vi "单数据解析_new.vi"(0 "Data1":u8, 1 "Data2":u8, 2 "Data3":u8, 3 "Data4":u8, 4 "Data5":u8, 5 "Data6":u8, 6 "Data7":u8, 7 "Data8":u8, 8 "ID":i32 format="%x", 9 "选项卡数值":enum32{"单体电压", "单体温度", "单体内阻", "单体SOC"}(ring)) -> (20 "位置":i32[](array[numeric]), 22 "数据":dbl[](array[numeric]), 24 "放电均衡":i32[](array[numeric]), 25 "充电均衡":i32[](array[numeric]), 26 "PF":i32, 27 "均衡故障":dbl[](array[numeric]))   [LabVIEW 2013]
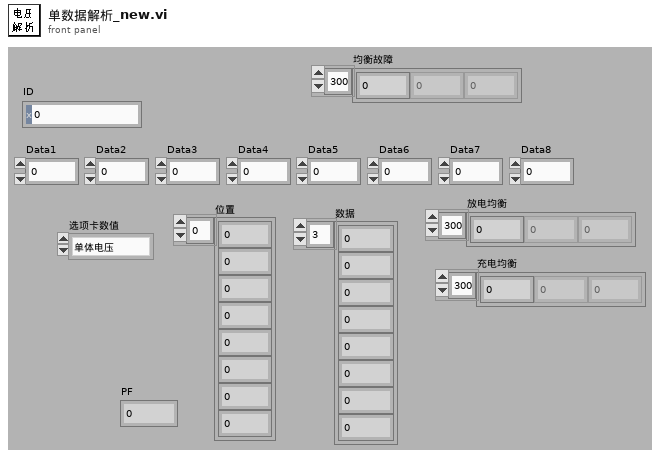
[diagram p1: front panel]
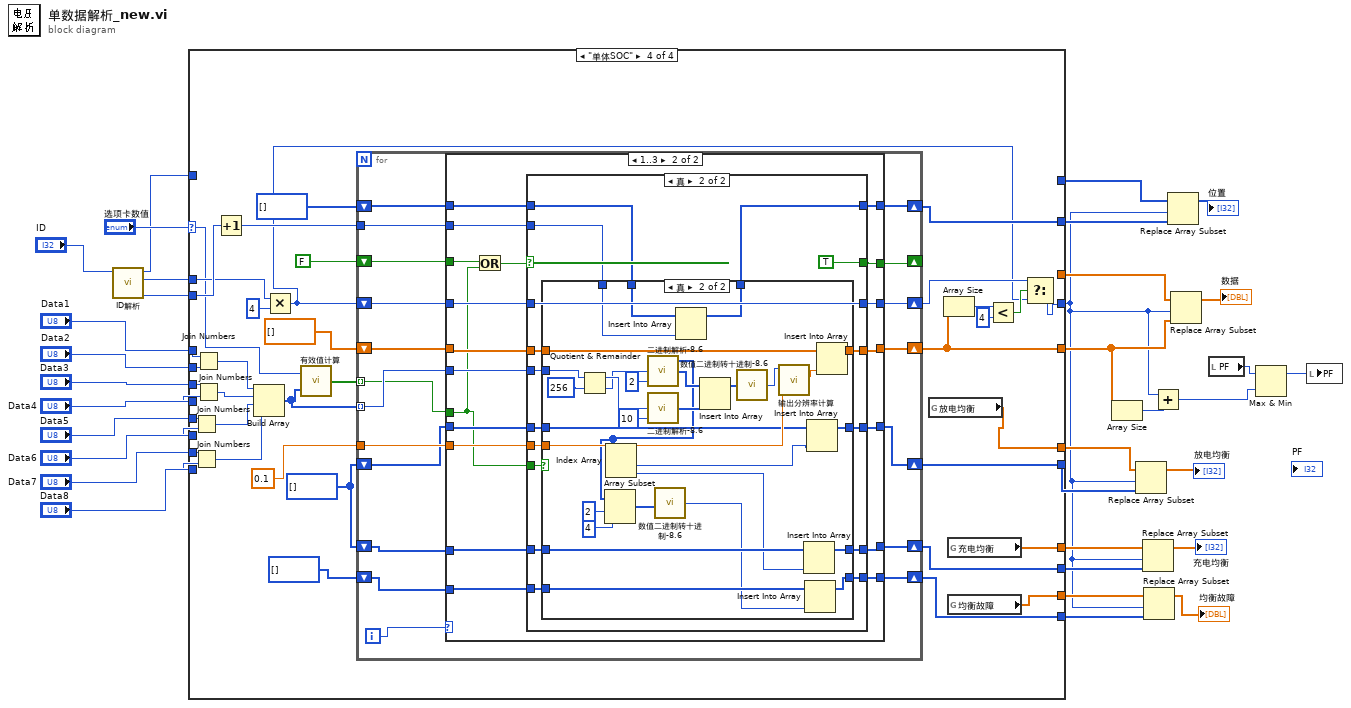
[diagram p0: block diagram]
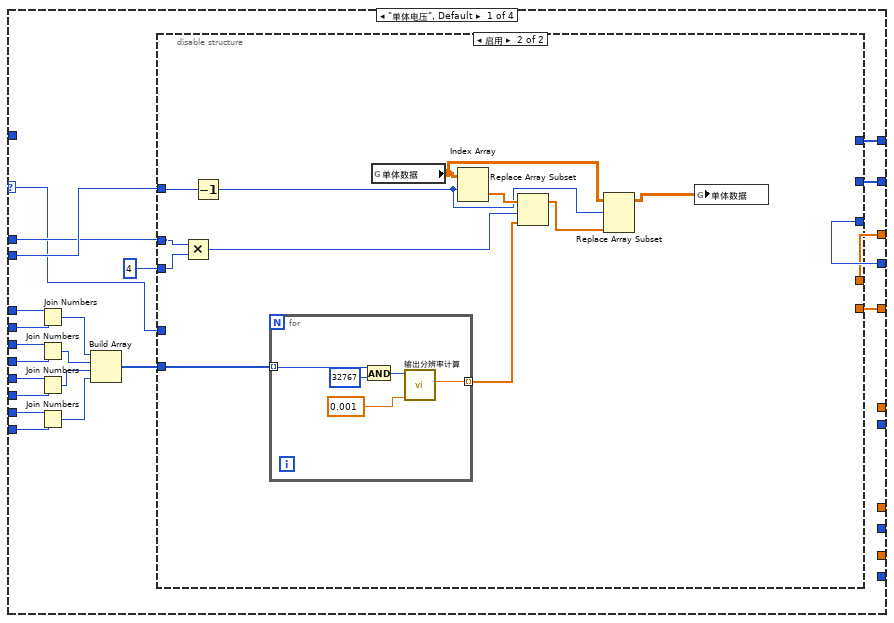
[diagram p2: hidden frame]
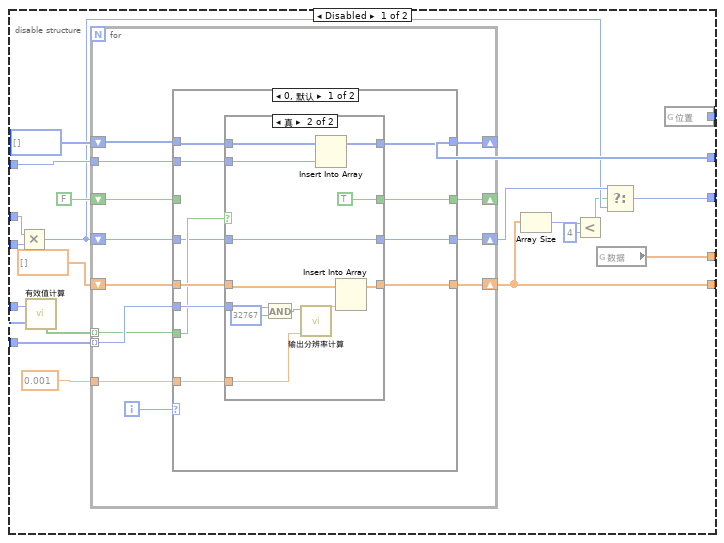
[diagram p3: hidden frame]
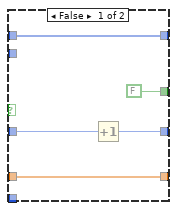
[diagram p4: hidden frame]
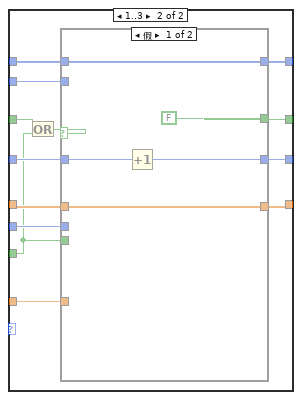
[diagram p5: hidden frame]
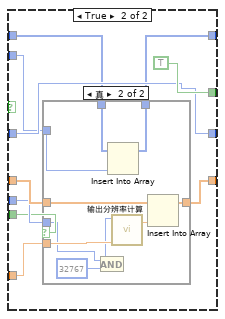
[diagram p6: hidden frame]
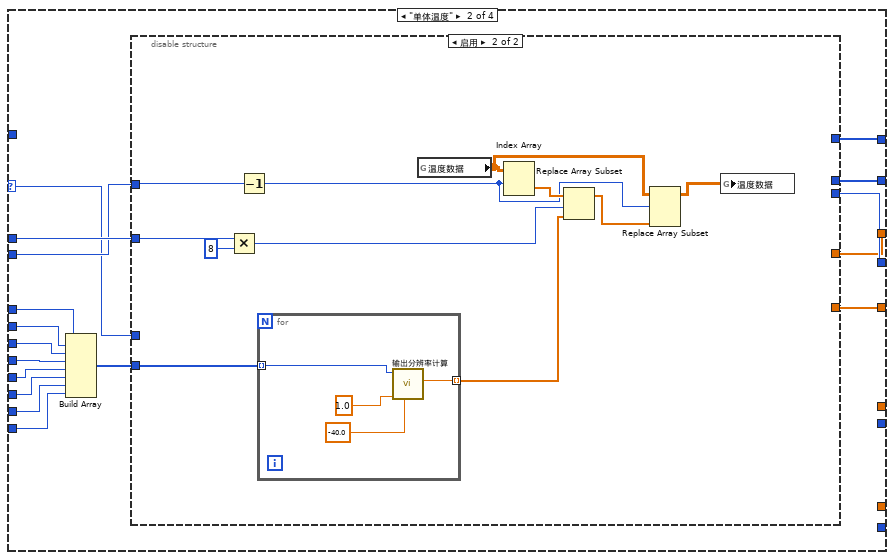
[diagram p8: hidden frame]
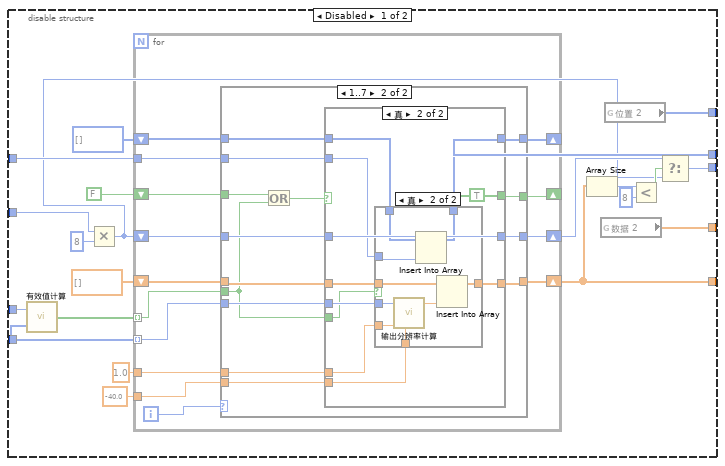
[diagram p9: hidden frame]
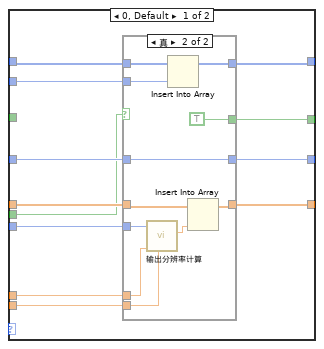
[diagram p10: hidden frame]
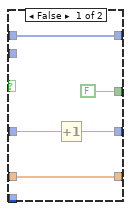
[diagram p11: hidden frame]
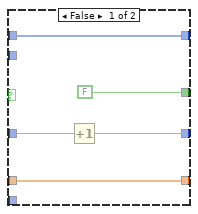
[diagram p12: hidden frame]
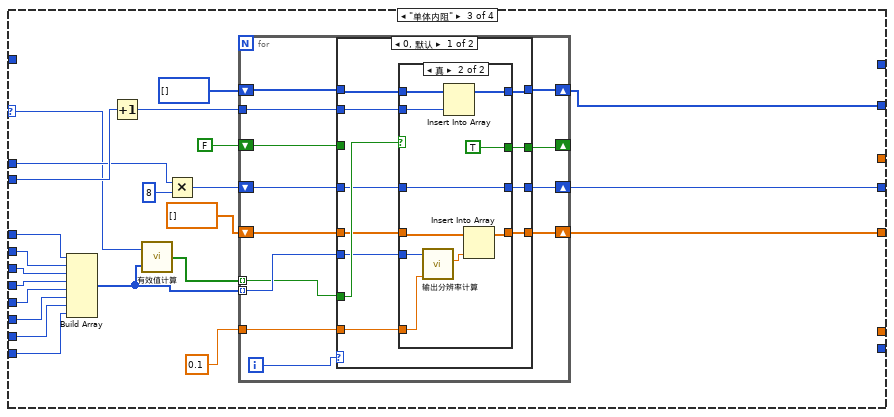
[diagram p14: hidden frame]
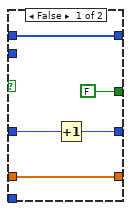
[diagram p15: hidden frame]
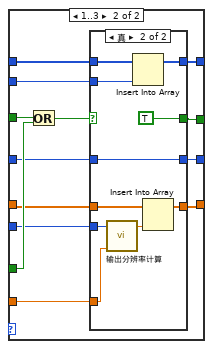
[diagram p16: hidden frame]
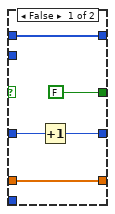
[diagram p17: hidden frame]
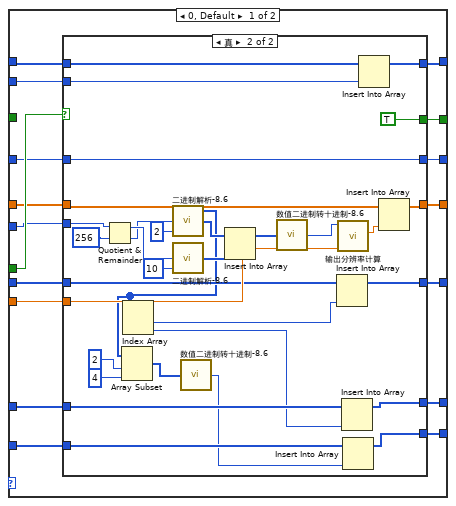
[diagram p18: hidden frame]
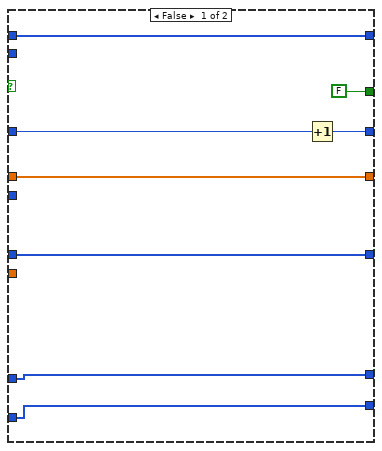
[diagram p19: hidden frame]
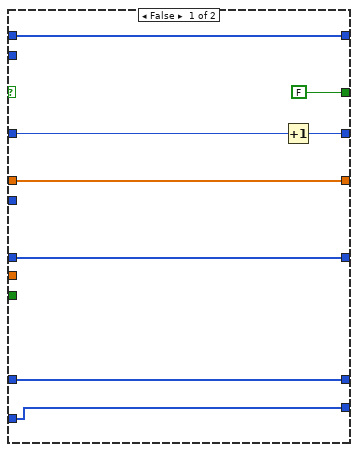
[diagram p20: hidden frame]
diagram:
  n1 = call "ID解析.vi"("ID"="ID") -> ("SA(4)"=w18:i32, "PF(2)"=w17:i32, "PDU(1)"=w29:i32)  [unwired: 8 out]
  n2 = case shown="\"单体SOC\"" "选项卡数值" {
    selector: "选项卡数值" -> [w34 w173 w310 w400]
    tunnel: "Data2" -> [w55 w187 w318 w429]
    tunnel: "Data1" -> [w54 w188 w319 w428]
    tunnel: "Data3" -> [w53 w186 w317 w427]
    tunnel: "Data4" -> [w52 w185 w316 w426]
    tunnel: "Data5" -> [w51 w184 w315 w425]
    tunnel: "Data7" -> [w50 w182 w313 w423]
    tunnel: "Data8" -> [w49 w181 w312 w422]
    tunnel: "Data6" -> [w48 w183 w314 w424]
    tunnel: [w46 w178 w328 w406] -> w3
    tunnel: [w47 w189 w323 w431] -> w33
    tunnel: [w45 w180 w322 w410] -> w5
    tunnel: w18 -> [w44 w177 w321 w430]
    tunnel: w17 -> [w43 w179 w320 w408]
    tunnel: [_ _ _ w417] -> w14
    tunnel: w29 -> [_ _ _ _]
    tunnel: [w37 w176 _ _] -> w16
    tunnel: [w36 w175 _ _] -> w15
    tunnel: [_ _ _ w416] -> w13
    tunnel: [_ _ _ w415] -> w12
    tunnel: [_ _ _ w405] -> w9
    tunnel: [_ _ _ w403] -> w8
    tunnel: [_ _ _ w402] -> w7
    frame "单体电压", Default {
      n3 = Join Numbers(hi=w54, lo=w55) -> ((hi.lo)=w41:u16)
      n4 = Join Numbers(hi=w53, lo=w52) -> ((hi.lo)=w40:u16)
      n5 = Join Numbers(hi=w51, lo=w48) -> ((hi.lo)=w39:u16)
      n6 = Join Numbers(hi=w50, lo=w49) -> ((hi.lo)=w38:u16)
      n7 = Build Array(w41, w40, w39, w38) -> (w35:u16[])
      n8 = disable-structure shown="启用" {
        disable-tunnel: [w75 _] -> w47
        disable-tunnel: [w74 _] -> w46
        disable-tunnel: [w73 _] -> w45
        disable-tunnel: w44 -> [w72 w166]
        disable-tunnel: w43 -> [w71 w164]
        disable-tunnel: 4 ("y") -> [w70 w163]
        disable-tunnel: [w60 _] -> w37
        disable-tunnel: [w59 _] -> w36
        disable-tunnel: w35 -> [w58 w167]
        disable-tunnel: w34 -> [w56 _]
        frame Disabled {
          n9 = Multiply(x=w71, y=w70) -> (x*y=w64:i32)
          n10 = call "有效值计算.vi"("数组"=w58, "选项卡数值"=w56) -> ("有效位"=w57:bool[])
          n11 = for {
            tunnel: w58 -> [w85] mode=indexing
            shift-right: [w86] -> w73
            shift-left: dbl[] [] -> [w87]
            tunnel: 0.001 ("分辨率") -> [w84]
            shift-right: [w82] -> w75
            shift-left: i32[] [] -> [w83]
            tunnel: w72 -> [w81]
            shift-right: [w80] -> _
            shift-left: FALSE -> [w79]
            shift-right: [w77] -> w65
            shift-left: w64 -> [w78]
            tunnel: w57 -> [w76] mode=indexing
            i -> [w88]
            n12 = case shown="0, 默认" w88 {
              tunnel: w76 -> [w91 w117]
              tunnel: [w99 w129] -> w80
              tunnel: w87 -> [w98 w128]
              tunnel: [w97 w127] -> w86
              tunnel: w85 -> [w96 w126]
              tunnel: w84 -> [w95 w125]
              tunnel: w83 -> [w94 w124]
              tunnel: [w93 w123] -> w82
              tunnel: w81 -> [w92 w122]
              tunnel: w79 -> [_ w118]
              tunnel: w78 -> [w90 w121]
              tunnel: [w89 w120] -> w77
              frame 0, Default {
                n13 = case shown="真" w91 {
                  tunnel: [FALSE TRUE] -> w99
                  tunnel: w98 -> [w103 w115]
                  tunnel: [w103 w114] -> w97
                  tunnel: w96 -> [_ w107]
                  tunnel: w95 -> [_ w112]
                  tunnel: w94 -> [w102 w111]
                  tunnel: [w102 w110] -> w93
                  tunnel: w92 -> [_ w109]
                  tunnel: w90 -> [w101 w108]
                  tunnel: [w100 w108] -> w89
                  frame False {
                    n14 = Increment(x=w101) -> (x+1=w100:i32)
                  }
                  frame True {
                    n15 = And(x=w107, y=u16 32767) -> (x .and. y?=w105:u16)
                    n16 = call "输出分辨率计算.vi"("分辨率"=w112, "数值 2"=w105) -> ("输出2"=w113:dbl)  [unwired: 4 in, 5 out]
                    n17 = Insert Into Array(array=w111, new element=w109) -> (w110:i32[])  [unwired: 1 in]
                    n18 = Insert Into Array(array=w115, new element=w113) -> (w114:dbl[])  [unwired: 1 in]
                  }
                }
              }
              frame 1..3 {
                n19 = Or(x=w118, y=w117) -> (x .or. y?=w119:bool)
                n20 = case shown="假" w119 {
                  tunnel: [FALSE TRUE] -> w129
                  tunnel: w128 -> [w134 w143]
                  tunnel: [w134 w142] -> w127
                  tunnel: w126 -> [_ w141]
                  tunnel: w125 -> [_ w140]
                  tunnel: w124 -> [w133 w136]
                  tunnel: [w133 w135] -> w123
                  tunnel: w122 -> [_ w137]
                  tunnel: w121 -> [w131 w139]
                  tunnel: [w130 w139] -> w120
                  tunnel: w117 -> [_ w138]
                  frame False {
                    n21 = Increment(x=w131) -> (x+1=w130:i32)
                  }
                  frame True {
                    n22 = case shown="真" w138 {
                      tunnel: w143 -> [w146 w156]
                      tunnel: [w146 w155] -> w142
                      tunnel: w141 -> [_ w148]
                      tunnel: w140 -> [_ w154]
                      tunnel: w137 -> [_ w152]
                      tunnel: w136 -> [w145 w151]
                      tunnel: [w145 w150] -> w135
                      frame False {
                      }
                      frame True {
                        n23 = And(x=w148, y=u16 32767) -> (x .and. y?=w147:u16)
                        n24 = Insert Into Array(array=w151, new element=w152) -> (w150:i32[])  [unwired: 1 in]
                        n25 = call "输出分辨率计算.vi"("分辨率"=w154, "数值 2"=w147) -> ("输出2"=w153:dbl)  [unwired: 4 in, 5 out]
                        n26 = Insert Into Array(array=w156, new element=w153) -> (w155:dbl[])  [unwired: 1 in]
                      }
                    }
                  }
                }
              }
            }
          }
          n27 = Array Size(array=w73) -> (size(s)=w63:i32)
          n28 = Less?(x=w63, y=4) -> (x < y?=w61:bool)
          n29 = global read "单体信息全局.vi" "数据"() -> (w59:dbl[])
          n30 = Select(t=w65, s=w61, f=w64) -> (s? t:f=w74:i32)
          n31 = global read "单体信息全局.vi" "位置"() -> (w60:i32[])
        }
        frame Enabled {
          n32 = Multiply(x=w164, y=w163) -> (x*y=w162:i32)
          n33 = Decrement(x=w166) -> (x-1=w159:i32)
          n34 = for {
            tunnel: w167 -> [w172] mode=indexing
            tunnel: [w168] -> w161 mode=indexing
            n35 = And(x=w172, y=u16 32767) -> (x .and. y?=w170:u16)
            n36 = call "输出分辨率计算.vi"("分辨率"=0.001, "数值 2"=w170) -> ("输出2"=w168:dbl)  [unwired: 4 in, 5 out]
          }
          n37 = global read "单体信息全局.vi" "单体数据"() -> (w160:dbl[][])
          n38 = Index Array(array=w160, index (row)=w159) -> (element=w165:dbl[])  [unwired: 1 in]
          n39 = Replace Array Subset(array=w165, new element=w161, index=w162) -> (w158:dbl[])
          n40 = Replace Array Subset(array=w160, new element=w158, index (row)=w159) -> (w157:dbl[][])  [unwired: 1 in]
          n41 = global write "单体信息全局.vi" "单体数据"(w157) -> ()
        }
      }
    }
    frame "单体温度" {
      n42 = Build Array(w188, w187, w186, w185, w184, w183, w182, w181) -> (w174:u8[])
      n43 = disable-structure shown="启用" {
        disable-tunnel: [w210 _] -> w189
        disable-tunnel: [w209 _] -> w180
        disable-tunnel: w179 -> [w208 w296]
        disable-tunnel: [w207 _] -> w178
        disable-tunnel: w177 -> [w206 w294]
        disable-tunnel: [w194 _] -> w176
        disable-tunnel: [w193 _] -> w175
        disable-tunnel: w174 -> [w192 w298]
        disable-tunnel: w173 -> [w190 _]
        frame Disabled {
          n44 = call "有效值计算.vi"("数组"=w192, "选项卡数值"=w190) -> ("有效位"=w191:bool[])
          n45 = Multiply(x=w208, y=8) -> (x*y=w195:i32)
          n46 = for {
            tunnel: w192 -> [w217] mode=indexing
            shift-right: [w222] -> w196
            shift-left: w195 -> [w223]
            shift-right: [w221] -> _
            shift-left: FALSE -> [w220]
            shift-right: [w218] -> w209
            shift-left: dbl[] [] -> [w219]
            tunnel: 1.0 ("分辨率") -> [w216]
            shift-right: [w214] -> w210
            shift-left: i32[] [] -> [w215]
            tunnel: w206 -> [w213]
            tunnel: -40.0 ("分辨率") -> [w212]
            tunnel: w191 -> [w211] mode=indexing
            i -> [w224]
            n47 = case shown="1..7" w224 {
              tunnel: w223 -> [w236 w264]
              tunnel: [w235 w263] -> w222
              tunnel: [w234 w262] -> w221
              tunnel: w220 -> [_ w265]
              tunnel: w219 -> [w233 w261]
              tunnel: [w232 w260] -> w218
              tunnel: w217 -> [w231 w259]
              tunnel: w216 -> [w230 w258]
              tunnel: w215 -> [w229 w257]
              tunnel: [w228 w256] -> w214
              tunnel: w213 -> [w227 w255]
              tunnel: w212 -> [w226 w254]
              tunnel: w211 -> [w225 w253]
              frame 0, Default {
                n48 = case shown="真" w225 {
                  tunnel: w236 -> [w240 w252]
                  tunnel: [w239 w252] -> w235
                  tunnel: [FALSE TRUE] -> w234
                  tunnel: w233 -> [w238 w250]
                  tunnel: [w238 w249] -> w232
                  tunnel: w231 -> [_ w248]
                  tunnel: w230 -> [_ w246]
                  tunnel: w229 -> [w237 w245]
                  tunnel: [w237 w244] -> w228
                  tunnel: w227 -> [_ w243]
                  tunnel: w226 -> [_ w242]
                  frame False {
                    n49 = Increment(x=w240) -> (x+1=w239:i32)
                  }
                  frame True {
                    n50 = call "输出分辨率计算.vi"("偏移量"=w242, "分辨率"=w246, "数值 2"=w248) -> ("输出2"=w247:dbl)  [unwired: 3 in, 5 out]
                    n51 = Insert Into Array(array=w245, new element=w243) -> (w244:i32[])  [unwired: 1 in]
                    n52 = Insert Into Array(array=w250, new element=w247) -> (w249:dbl[])  [unwired: 1 in]
                  }
                }
              }
              frame 1..7 {
                n53 = Or(x=w265, y=w253) -> (x .or. y?=w266:bool)
                n54 = case shown="真" w266 {
                  tunnel: w264 -> [w271 w282]
                  tunnel: [w270 w282] -> w263
                  tunnel: [FALSE TRUE] -> w262
                  tunnel: w261 -> [w268 w280]
                  tunnel: [w268 w279] -> w260
                  tunnel: w259 -> [_ w278]
                  tunnel: w258 -> [_ w277]
                  tunnel: w257 -> [w267 w274]
                  tunnel: [w267 w273] -> w256
                  tunnel: w255 -> [_ w275]
                  tunnel: w254 -> [_ w276]
                  tunnel: w253 -> [_ w272]
                  frame False {
                    n55 = Increment(x=w271) -> (x+1=w270:i32)
                  }
                  frame True {
                    n56 = case shown="真" w272 {
                      tunnel: w280 -> [w284 w293]
                      tunnel: [w284 w292] -> w279
                      tunnel: w278 -> [_ w291]
                      tunnel: w277 -> [_ w290]
                      tunnel: w276 -> [_ w289]
                      tunnel: w275 -> [_ w287]
                      tunnel: w274 -> [w283 w286]
                      tunnel: [w283 w285] -> w273
                      frame False {
                      }
                      frame True {
                        n57 = call "输出分辨率计算.vi"("偏移量"=w289, "分辨率"=w290, "数值 2"=w291) -> ("输出2"=w288:dbl)  [unwired: 3 in, 5 out]
                        n58 = Insert Into Array(array=w286, new element=w287) -> (w285:i32[])  [unwired: 1 in]
                        n59 = Insert Into Array(array=w293, new element=w288) -> (w292:dbl[])  [unwired: 1 in]
                      }
                    }
                  }
                }
              }
            }
          }
          n60 = Array Size(array=w209) -> (size(s)=w199:i32)
          n61 = global read "单体信息全局.vi" "数据 2"() -> (w193:dbl[])
          n62 = global read "单体信息全局.vi" "位置 2"() -> (w194:i32[])
          n63 = Less?(x=w199, y=8) -> (x < y?=w197:bool)
          n64 = Select(t=w196, s=w197, f=w195) -> (s? t:f=w207:i32)
        }
        frame Enabled {
          n65 = Multiply(x=w296, y=8) -> (x*y=w303:i32)
          n66 = Decrement(x=w294) -> (x-1=w300:i32)
          n67 = for {
            tunnel: w298 -> [w305] mode=indexing
            tunnel: [w307] -> w302 mode=indexing
            n68 = call "输出分辨率计算.vi"("偏移量"=sgl -40.0, "分辨率"=1.0, "数值 2"=w305) -> ("输出2"=w307:dbl)  [unwired: 3 in, 5 out]
          }
          n69 = global read "单体信息全局.vi" "温度数据"() -> (w301:sgl[][])
          n70 = Index Array(array=w301, index (row)=w300) -> (element=w304:sgl[])  [unwired: 1 in]
          n71 = Replace Array Subset(array=w304, new element=w302, index=w303) -> (w299:sgl[])
          n72 = Replace Array Subset(array=w301, new element=w299, index (row)=w300) -> (w297:sgl[][])  [unwired: 1 in]
          n73 = global write "单体信息全局.vi" "温度数据"(w297) -> ()
        }
      }
    }
    frame "单体内阻" {
      n74 = Build Array(w319, w318, w317, w316, w315, w314, w313, w312) -> (w311:u8[])
      n75 = Increment(x=w321) -> (x+1=w325:i32)
      n76 = call "有效值计算.vi"("数组"=w311, "选项卡数值"=w310) -> ("有效位"=w309:bool[])
      n77 = Multiply(x=w320, y=8) -> (x*y=w330:i32)
      n78 = for {
        tunnel: w311 -> [w337] mode=indexing
        shift-right: [w342] -> w328
        shift-left: w330 -> [w343]
        shift-right: [w341] -> _
        shift-left: FALSE -> [w340]
        shift-right: [w338] -> w322
        shift-left: dbl[] [] -> [w339]
        tunnel: 0.1 ("分辨率") -> [w336]
        shift-right: [w334] -> w323
        shift-left: i32[] [] -> [w335]
        tunnel: w325 -> [w333]
        tunnel: w309 -> [w332] mode=indexing
        i -> [w344]
        n79 = case shown="0, 默认" w344 {
          tunnel: w332 -> [w355 w381]
          tunnel: w343 -> [w354 w380]
          tunnel: [w353 w379] -> w342
          tunnel: [w352 w378] -> w341
          tunnel: w340 -> [_ w382]
          tunnel: w339 -> [w351 w377]
          tunnel: [w350 w376] -> w338
          tunnel: w337 -> [w349 w375]
          tunnel: w336 -> [w348 w374]
          tunnel: w335 -> [w347 w373]
          tunnel: [w346 w372] -> w334
          tunnel: w333 -> [w345 w371]
          frame 0, Default {
            n80 = case shown="真" w355 {
              tunnel: w354 -> [w359 w370]
              tunnel: [w358 w370] -> w353
              tunnel: [FALSE TRUE] -> w352
              tunnel: w351 -> [w357 w368]
              tunnel: [w357 w367] -> w350
              tunnel: w349 -> [_ w366]
              tunnel: w348 -> [_ w364]
              tunnel: w347 -> [w356 w363]
              tunnel: [w356 w362] -> w346
              tunnel: w345 -> [_ w361]
              frame False {
                n81 = Increment(x=w359) -> (x+1=w358:i32)
              }
              frame True {
                n82 = call "输出分辨率计算.vi"("分辨率"=w364, "数值 2"=w366) -> ("输出2"=w365:dbl)  [unwired: 4 in, 5 out]
                n83 = Insert Into Array(array=w363, new element=w361) -> (w362:i32[])  [unwired: 1 in]
                n84 = Insert Into Array(array=w368, new element=w365) -> (w367:dbl[])  [unwired: 1 in]
              }
            }
          }
          frame 1..3 {
            n85 = Or(x=w382, y=w381) -> (x .or. y?=w383:bool)
            n86 = case shown="真" w383 {
              tunnel: w380 -> [w388 w398]
              tunnel: [w387 w398] -> w379
              tunnel: [FALSE TRUE] -> w378
              tunnel: w377 -> [w385 w396]
              tunnel: [w385 w395] -> w376
              tunnel: w375 -> [_ w394]
              tunnel: w374 -> [_ w392]
              tunnel: w373 -> [w384 w391]
              tunnel: [w384 w390] -> w372
              tunnel: w371 -> [_ w389]
              frame False {
                n87 = Increment(x=w388) -> (x+1=w387:i32)
              }
              frame True {
                n88 = call "输出分辨率计算.vi"("分辨率"=w392, "数值 2"=w394) -> ("输出2"=w393:dbl)  [unwired: 4 in, 5 out]
                n89 = Insert Into Array(array=w391, new element=w389) -> (w390:i32[])  [unwired: 1 in]
                n90 = Insert Into Array(array=w396, new element=w393) -> (w395:dbl[])  [unwired: 1 in]
              }
            }
          }
        }
      }
    }
    frame "单体SOC" {
      w414 = i32[] []
      n91 = Join Numbers(hi=w425, lo=w424) -> ((hi.lo)=w420:u16)
      n92 = Join Numbers(hi=w423, lo=w422) -> ((hi.lo)=w421:u16)
      n93 = Join Numbers(hi=w428, lo=w429) -> ((hi.lo)=w418:u16)
      n94 = Join Numbers(hi=w427, lo=w426) -> ((hi.lo)=w419:u16)
      n95 = Increment(x=w430) -> (x+1=w433:i32)
      n96 = Build Array(w418, w419, w420, w421) -> (w401:u16[])
      n97 = Multiply(x=w408, y=4) -> (x*y=w407:i32)
      n98 = call "有效值计算.vi"("数组"=w401, "选项卡数值"=w400) -> ("有效位"=w399:bool[])
      n99 = for {
        tunnel: w401 -> [w443] mode=indexing
        shift-right: [w454] -> w409
        shift-left: w407 -> [w455]
        shift-right: [w453] -> _
        shift-left: FALSE -> [w452]
        shift-right: [w450] -> w410
        shift-left: dbl[] [] -> [w451]
        tunnel: 0.1 ("分辨率") -> [w449]
        shift-right: [w447] -> w431
        shift-left: i32[] [] -> [w448]
        tunnel: w433 -> [w446]
        shift-right: [w444] -> w417
        shift-left: w414 -> [w445]
        shift-right: [w441] -> w405
        shift-left: w414 -> [w442]
        shift-right: [w439] -> w403
        shift-left: i32[] [] -> [w440]
        tunnel: w399 -> [w438] mode=indexing
        i -> [w456]
        n100 = case shown="1..3" w456 {
          tunnel: w438 -> [w473 w514]
          tunnel: w455 -> [w472 w530]
          tunnel: [w471 w529] -> w454
          tunnel: [w470 w528] -> w453
          tunnel: w452 -> [_ w531]
          tunnel: w451 -> [w469 w527]
          tunnel: [w468 w526] -> w450
          tunnel: w443 -> [w461 w525]
          tunnel: w449 -> [w467 w524]
          tunnel: w448 -> [w466 w523]
          tunnel: [w465 w522] -> w447
          tunnel: w446 -> [w464 w521]
          tunnel: [w463 w519] -> w444
          tunnel: w445 -> [w462 w520]
          tunnel: w442 -> [w460 w518]
          tunnel: [w459 w517] -> w441
          tunnel: w440 -> [w458 w516]
          tunnel: [w457 w515] -> w439
          frame 0, Default {
            n101 = case shown="真" w473 {
              tunnel: w472 -> [w480 w513]
              tunnel: [w479 w513] -> w471
              tunnel: [FALSE TRUE] -> w470
              tunnel: w469 -> [w478 w511]
              tunnel: [w478 w510] -> w468
              tunnel: w467 -> [_ w508]
              tunnel: w466 -> [w477 w507]
              tunnel: [w477 w506] -> w465
              tunnel: w464 -> [_ w505]
              tunnel: [w476 w504] -> w463
              tunnel: w462 -> [w476 w503]
              tunnel: w461 -> [_ w495]
              tunnel: w460 -> [w475 w493]
              tunnel: [w475 w492] -> w459
              tunnel: w458 -> [w474 w485]
              tunnel: [w474 w484] -> w457
              frame False {
                n102 = Increment(x=w480) -> (x+1=w479:i32)
              }
              frame True {
                n103 = Quotient & Remainder(x=w495, y=u16 256) -> (x-y*floor(x/y)=w501:u16, floor(x/y)=w500:u16)
                n104 = call "二进制解析-8.6.vi"("索引"=2, "数值"=w500) -> ("低位子数组"=w498:i32[], "高位子数组"=w488:i32[])  [unwired: 2 out]
                n105 = Array Subset(array=w488, index=2 ("索引"), length=4 ("长度")) -> (w483:i32[])
                n106 = Index Array(array=w488) -> (element #1=w491:i32, element #2=w490:i32)  [unwired: 2 in]
                n107 = call "二进制解析-8.6.vi"("索引"=10, "数值"=w501) -> ("低位子数组"=w497:i32[])  [unwired: 3 out]
                n108 = call "数值二进制转十进制-8.6.vi"("子数组"=w483) -> ("十进制数值"=w482:i32)  [unwired: 4 out]
                n109 = Insert Into Array(array=w498, new element=w497) -> (w496:i32[])  [unwired: 1 in]
                n110 = call "数值二进制转十进制-8.6.vi"("子数组"=w496) -> ("十进制数值"=w494:i32)  [unwired: 4 out]
                n111 = Insert Into Array(array=w503, new element=w491) -> (w504:i32[])  [unwired: 1 in]
                n112 = call "输出分辨率计算.vi"("分辨率"=w508, "数值 2"=w494) -> ("输出2"=w509:dbl)  [unwired: 4 in, 5 out]
                n113 = Insert Into Array(array=w493, new element=w490) -> (w492:i32[])  [unwired: 1 in]
                n114 = Insert Into Array(array=w485, new element=w482) -> (w484:i32[])  [unwired: 1 in]
                n115 = Insert Into Array(array=w507, new element=w505) -> (w506:i32[])  [unwired: 1 in]
                n116 = Insert Into Array(array=w511, new element=w509) -> (w510:dbl[])  [unwired: 1 in]
              }
            }
          }
          frame 1..3 {
            n117 = Or(x=w531, y=w514) -> (x .or. y?=w532:bool)
            n118 = case shown="真" w532 {
              tunnel: w530 -> [w540 w556]
              tunnel: [w539 w556] -> w529
              tunnel: [FALSE TRUE] -> w528
              tunnel: w527 -> [w537 w554]
              tunnel: [w537 w553] -> w526
              tunnel: w525 -> [_ w549]
              tunnel: w524 -> [_ w552]
              tunnel: w523 -> [w536 w543]
              tunnel: [w536 w541] -> w522
              tunnel: w521 -> [_ w542]
              tunnel: w520 -> [w535 w551]
              tunnel: [w535 w550] -> w519
              tunnel: w518 -> [w534 w548]
              tunnel: [w534 w547] -> w517
              tunnel: w516 -> [w533 w546]
              tunnel: [w533 w545] -> w515
              tunnel: w514 -> [_ w544]
              frame False {
                n119 = Increment(x=w540) -> (x+1=w539:i32)
              }
              frame True {
                n120 = case shown="真" w544 {
                  tunnel: w554 -> [w561 w591]
                  tunnel: [w561 w590] -> w553
                  tunnel: w552 -> [_ w589]
                  tunnel: w551 -> [w560 w588]
                  tunnel: [w560 w587] -> w550
                  tunnel: w549 -> [_ w586]
                  tunnel: w548 -> [w559 w585]
                  tunnel: [w559 w584] -> w547
                  tunnel: w546 -> [w558 w583]
                  tunnel: [w558 w582] -> w545
                  tunnel: w543 -> [w557 w564]
                  tunnel: w542 -> [_ w563]
                  tunnel: [w557 w562] -> w541
                  frame False {
                  }
                  frame True {
                    n121 = Quotient & Remainder(x=w586, y=u16 256) -> (x-y*floor(x/y)=w578:u16, floor(x/y)=w577:u16)
                    n122 = call "二进制解析-8.6.vi"("索引"=2, "数值"=w577) -> ("低位子数组"=w575:i32[], "高位子数组"=w570:i32[])  [unwired: 2 out]
                    n123 = Array Subset(array=w570, index=2 ("索引"), length=4 ("长度")) -> (w566:i32[])
                    n124 = Index Array(array=w570) -> (element #1=w569:i32, element #2=w571:i32)  [unwired: 2 in]
                    n125 = call "二进制解析-8.6.vi"("索引"=10, "数值"=w578) -> ("低位子数组"=w574:i32[])  [unwired: 3 out]
                    n126 = call "数值二进制转十进制-8.6.vi"("子数组"=w566) -> ("十进制数值"=w565:i32)  [unwired: 4 out]
                    n127 = Insert Into Array(array=w564, new element=w563) -> (w562:i32[])  [unwired: 1 in]
                    n128 = Insert Into Array(array=w575, new element=w574) -> (w573:i32[])  [unwired: 1 in]
                    n129 = call "数值二进制转十进制-8.6.vi"("子数组"=w573) -> ("十进制数值"=w572:i32)  [unwired: 4 out]
                    n130 = call "输出分辨率计算.vi"("分辨率"=w589, "数值 2"=w572) -> ("输出2"=w581:dbl)  [unwired: 4 in, 5 out]
                    n131 = Insert Into Array(array=w585, new element=w571) -> (w584:i32[])  [unwired: 1 in]
                    n132 = Insert Into Array(array=w583, new element=w565) -> (w582:i32[])  [unwired: 1 in]
                    n133 = Insert Into Array(array=w588, new element=w569) -> (w587:i32[])  [unwired: 1 in]
                    n134 = Insert Into Array(array=w591, new element=w581) -> (w590:dbl[])  [unwired: 1 in]
                  }
                }
              }
            }
          }
        }
      }
      n135 = global read "单体信息全局.vi" "放电均衡"() -> (w416:dbl[])
      n136 = Array Size(array=w410) -> (size(s)=w413:i32)
      n137 = global read "单体信息全局.vi" "充电均衡"() -> (w415:dbl[])
      n138 = global read "单体信息全局.vi" "均衡故障"() -> (w402:dbl[])
      n139 = Less?(x=w413, y=4) -> (x < y?=w411:bool)
      n140 = Select(t=w409, s=w411, f=w407) -> (s? t:f=w406:i32)
    }
  }
  n141 = Array Size(array=w5) -> (size(s)=w4:i32)
  n142 = Replace Array Subset(array=w13, new element=w14, index=w3) -> (→"放电均衡":dbl[])
  n143 = Replace Array Subset(array=w12, new element=w9, index=w3) -> (→"充电均衡":dbl[])
  n144 = Replace Array Subset(array=w7, new element=w8, index=w3) -> (→"均衡故障":dbl[])
  n145 = Add(x=w3, y=w4) -> (x+y=w2:i32)
  n146 = Replace Array Subset(array=w16, new element=w33, index=w3) -> (→"位置":i32[])
  n147 = Replace Array Subset(array=w15, new element=w5, index=w3) -> (→"数据":dbl[])
  n148 = local read "PF"() -> (w28:i32)
  n149 = Max & Min(x=w28, y=w2) -> (max(x,y)=w1:i32)  [unwired: 1 out]
  n150 = local write "PF"(w1) -> ()
